vi "demo - wf chart.vi"() -> ()   [LabVIEW 2024]
doc: "#vi_description \nPlot a random number onto a waveform chart\nThetic Engineering Ltd."
panel:
  in  "Stop":bool
  out "alarm":bool
  in  "threshold":dbl(knob)=0.49568843009143065 min=0.1 step=0.1 scale=0.1..0.9
  out "Waveform Chart":cluster{"number: 0 to 1":dbl, "threshold":dbl}(graph)
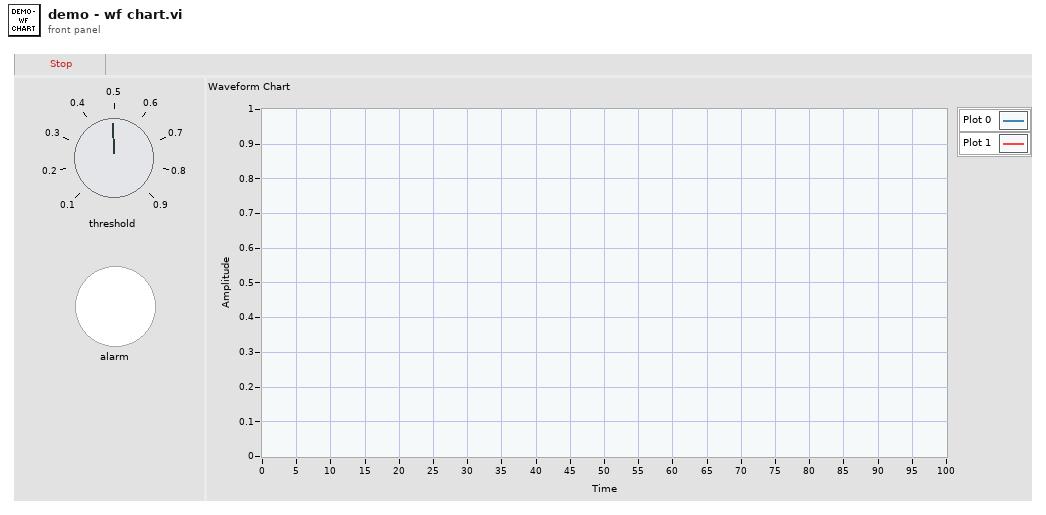
[diagram p1: front panel]
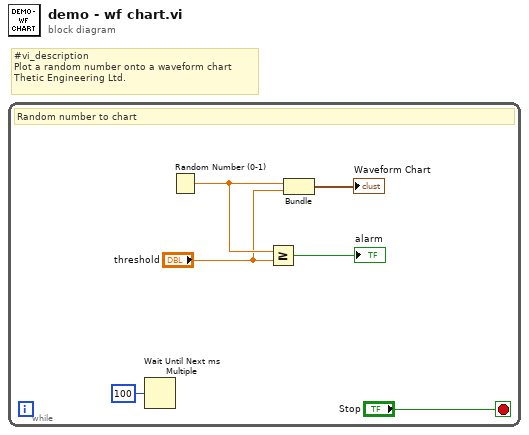
[diagram p0: block diagram]
diagram:
  # "#vi_description \nPlot a random number onto a waveform chart\nThetic Engineering Ltd."
  n1 = while {
    stop <- "Stop" stop-if-true
    # "Random number to chart"
    n2 = Wait Until Next ms Multiple(millisecond multiple=u32 100) -> ()  [unwired: 1 out]
    n3 = Random Number (0-1)() -> (number: 0 to 1=w4:dbl)
    n4 = Greater Or Equal?(x=w4, y="threshold") -> (x >= y?=→"alarm":bool)
    n5 = Bundle("number: 0 to 1"=w4, "threshold"="threshold") -> (→"Waveform Chart":cluster{"number: 0 to 1":dbl, "threshold":dbl})  [unwired: 1 in]
  }
